vi "pause_zero_bit.vi"(1 "Входная последовательность":dbl[](array[numeric])) -> (0 "Массив с паузами":dbl[](array[numeric]))   [LabVIEW 2017]
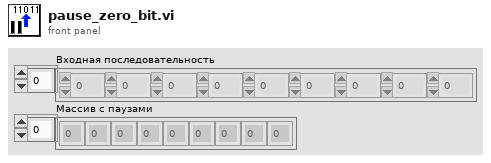
[diagram p1: front panel]
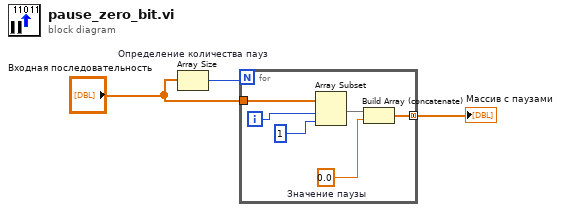
[diagram p0: block diagram]
diagram:
  n1 = Array Size "Определение количества пауз"(array="Входная последовательность") -> (size(s)=w3:i32)
  n2 = for {
    N: w3 -> [_]
    tunnel: "Входная последовательность" -> [w6]
    tunnel: [w5] -> w2 mode=concatenating
    i -> [w4]
    w7 = 0.0  # Значение паузы
    n3 = Array Subset(array=w6, index=w4, length=1) -> (w8:dbl[])
    n4 = Build Array (concatenate)(w8, w7) -> (w5:dbl[])
  }
  "Массив с паузами" <- w2
